vi "setUp.vi"(8 "error in (no error)":errorcluster, 11 "LUnit test in":refnum<class "LUnit Test 16.lvclass">) -> (0 "error out":errorcluster, 3 "LUnit test out":refnum<class "LUnit Test 16.lvclass">)   [LabVIEW 2020, in "LUnit Test 16.lvclass"]
uses:
  LUnit Test 16.lvclass
  <vilib>/Asteme/LUnit/Test Case.lvclass
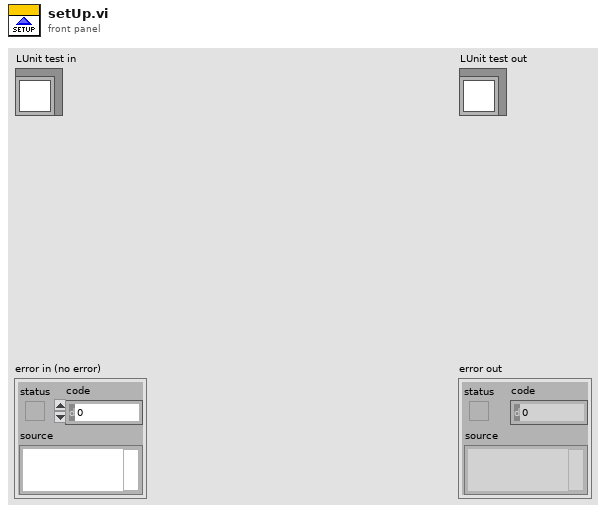
[diagram p1: front panel]
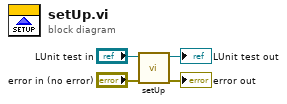
[diagram p0: block diagram]
diagram:
  n1 = call-parent "setUp.vi"("error in (no error)"="error in (no error)", "LUnit Test Case In"="LUnit test in") -> ("error out"=→"error out":errorcluster, "LUnit Test Case Out"=→"LUnit test out":refnum<class "LUnit Test 16.lvclass">)  [unwired: 8 in]
